vi "macro_MathUtils_ClampInput.vi"   [LabVIEW 2019, in "Trajectory_Library.lvlib"]
uses:
  Trajectory_Library.lvlib
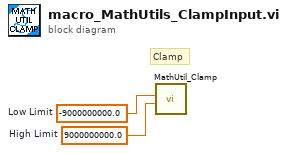
[diagram p0: block diagram]
diagram:
  w1 = 9000000000.0  # High Limit
  w2 = -9000000000.0  # Low Limit
  # "Clamp"
  n1 = call "MathUtil_Clamp.vi"("High Limit"=w1, "Low Limit"=w2) -> ()  [unwired: 9 in, 1 out]
